vi "Global.vi"() -> ()   [LabVIEW 2019]
panel:
  in  "String":string
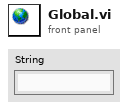
[diagram p1: front panel]
diagram:
